vi "T_step_VTI.vi"   [LabVIEW 2019]
uses:
  Global/Global Variables/global.vi
  Instrument_Setup.vi
  Global/Global Variables/Data_Display_global.vi
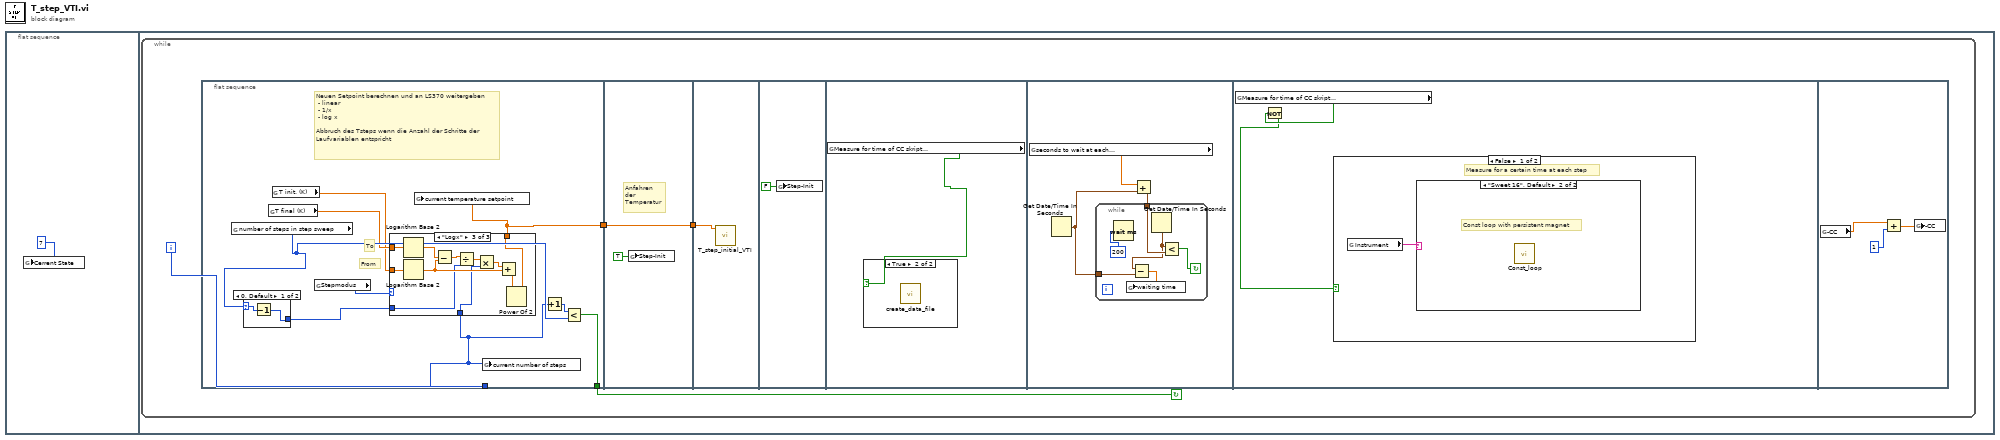
[diagram p0: block diagram]
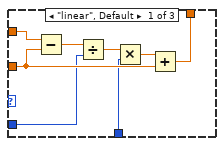
[diagram p3: hidden frame]
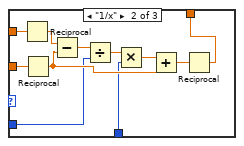
[diagram p4: hidden frame]
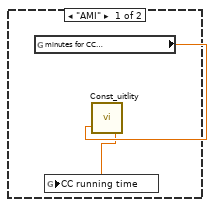
[diagram p6: hidden frame]
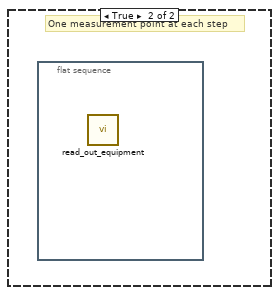
[diagram p7: hidden frame]
diagram:
  n1 = flat-sequence {
    frame #0 {
      n2 = global write "global.vi" "Cerrent State"(7) -> ()
    }
    frame #1 {
      n3 = while {
        i -> [w5]
        stop <- w4 continue-if-true
        n4 = flat-sequence {
          tunnel: w5 -> [w7]
          tunnel: [w8] -> w4
          tunnel: [w6] -> w2
          tunnel: [w48] -> w3
          tunnel: w2 -> [w48]
          tunnel: w3 -> [w50]
          frame #0 {
            # "Neuen Setpoint berechnen und an LS370 weitergeben\n - linear\n - 1/x\n - log x\n\nAbbruch des Tsteps wenn die Anzahl der Schritte der \nLaufvariablen entspricht"
            # "From"
            # "To"
            n5 = global read "global.vi" "number of steps in step sweep"() -> (w12:i32)
            n6 = case shown="0, Default" w12 {
              selector: w12 -> [w16 w17]
              tunnel: [w15 w17] -> w13
              frame 0, Default {
                n7 = Decrement(x=w16) -> (x-1=w15:i32)
              }
              frame 1 {
              }
            }
            n8 = global read "global.vi" "T final (K)"() -> (w10:dbl)
            n9 = global read "global.vi" "T init. (K)"() -> (w9:dbl)
            n10 = global read "Instrument_Setup.vi" "Stepmodus"() -> (w11:enum16{"linear", "1/x", "Logx"})
            n11 = case shown="\"Logx\"" w11 {
              tunnel: w10 -> [w25 w35 w47]
              tunnel: w9 -> [w22 w36 w46]
              tunnel: [w20 w30 w39] -> w6
              tunnel: w13 -> [w19 w27 w38]
              tunnel: w7 -> [w18 w26 w37]
              frame "linear", Default {
                n12 = Subtract(x=w25, y=w22) -> (x-y=w24:dbl)
                n13 = Divide(x=w24, y=w19) -> (x/y=w23:dbl)
                n14 = Multiply(x=w23, y=w18) -> (x*y=w21:dbl)
                n15 = Add(x=w21, y=w22) -> (x+y=w20:dbl)
              }
              frame "1/x" {
                n16 = Reciprocal(x=w35) -> (1/x=w29:dbl)
                n17 = Reciprocal(x=w36) -> (1/x=w28:dbl)
                n18 = Subtract(x=w29, y=w28) -> (x-y=w34:dbl)
                n19 = Divide(x=w34, y=w27) -> (x/y=w33:dbl)
                n20 = Multiply(x=w33, y=w26) -> (x*y=w32:dbl)
                n21 = Add(x=w32, y=w28) -> (x+y=w31:dbl)
                n22 = Reciprocal(x=w31) -> (1/x=w30:dbl)
              }
              frame "Logx" {
                n23 = Logarithm Base 2(1:w47) -> (0:w45:dbl)
                n24 = Logarithm Base 2(1:w46) -> (0:w41:dbl)
                n25 = Subtract(x=w45, y=w41) -> (x-y=w44:dbl)
                n26 = Divide(x=w44, y=w38) -> (x/y=w43:dbl)
                n27 = Multiply(x=w43, y=w37) -> (x*y=w42:dbl)
                n28 = Add(x=w42, y=w41) -> (x+y=w40:dbl)
                n29 = Power Of 2(x=w40) -> (2^x=w39:dbl)
              }
            }
            n30 = global write "Data_Display_global.vi" "current temperature setpoint"(w6) -> ()
            n31 = global write "Data_Display_global.vi" "current number of steps"(w7) -> ()
            n32 = Increment(x=w7) -> (x+1=w14:i32)
            n33 = Less?(x=w14, y=w12) -> (x < y?=w8:bool)
          }
          frame #1 {
            # "Anfahren \nder \nTemperatur"
            n34 = global write "global.vi" "Step-Init"(TRUE) -> ()
          }
          frame #2 {
            n35 = call "T_step_initial_VTI.vi"("Current Step Setpoint"=w50) -> ()  [unwired: 11 in]
          }
          frame #3 {
            n36 = global write "global.vi" "Step-Init"(FALSE) -> ()
          }
          frame #4 {
            n37 = global read "Instrument_Setup.vi" "Measure for time of CC skript\nat each field step point"() -> (w52:bool)
            n38 = case shown="True" w52 {
              frame False {
              }
              frame True {
                n39 = call "create_data_file.vi"() -> ()  [unwired: 3 in]
              }
            }
          }
          frame #5 {
            n40 = global read "Instrument_Setup.vi" "seconds to wait at each\nfield step in a step sweep"() -> (w53:dbl)
            n41 = Get Date/Time In Seconds() -> (seconds since 1Jan1904=w54:timestamp)
            n42 = Add(x=w53, y=w54) -> (x+y=w55:timestamp)
            n43 = while {
              tunnel: w55 -> [w61]
              tunnel: w54 -> [w57]
              stop <- w60 continue-if-true
              n44 = Wait (ms)(milliseconds to wait=u32 200) -> ()  [unwired: 1 out]
              n45 = Get Date/Time In Seconds() -> (seconds since 1Jan1904=w58:timestamp)
              n46 = Subtract(x=w58, y=w57) -> (x-y=w56:dbl)
              n47 = global write "Data_Display_global.vi" "waiting time"(w56) -> ()
              n48 = Less?(x=w58, y=w61) -> (x < y?=w60:bool)
            }
          }
          frame #6 {
            n49 = global read "Instrument_Setup.vi" "Measure for time of CC skript\nat each field step point"() -> (w63:bool)
            n50 = Not(x=w63) -> (.not. x?=w62:bool)
            n51 = case shown="False" w62 {
              frame False {
                # "Measure for a certain time at each step"
                n52 = global read "Instrument_Setup.vi" "Instrument"() -> (w64:string)
                n53 = case shown="\"Sweet 16\", Default" w64 {
                  frame "AMI" {
                    n54 = global read "Instrument_Setup.vi" "minutes for CC\nto run"() -> (w66:dbl)
                    n55 = call "Const_uitlity.vi"("Duration"=w66) -> ("Minutes passed"=w65:dbl)  [unwired: 1 in]
                    n56 = global write "Data_Display_global.vi" "CC running time"(w65) -> ()
                  }
                  frame "Sweet 16", Default {
                    # "Const loop with persistent magnet"
                    n57 = call "Const_loop.vi"() -> ()  [unwired: 4 in]
                  }
                }
              }
              frame True {
                # "One measurement point at each step"
                n58 = flat-sequence {
                  frame #0 {
                    n59 = call "read_out_equipment.vi"() -> ()  [unwired: 1 in]
                  }
                }
              }
            }
          }
          frame #7 {
            n60 = global read "global.vi" "-CC"() -> (w69:dbl)
            n61 = Add(x=w69, y=1) -> (x+y=w67:dbl)
            n62 = global write "global.vi" "-CC"(w67) -> ()
          }
        }
      }
    }
  }
